vi "Fetch Measurement (Occupied Bandwidth).vi"(8 "error in (no error)":errorcluster, 9 "Timeout (20000 ms)":i32=20000, 11 "VISA resource name":refnum<visa-resource-name>) -> (0 "error out":errorcluster, 1 "Occupied Bandwidth (Hz)":dbl format="%#.6g", 2 "Transmit Frequency Error (Hz)":dbl format="%#.6g", 3 "VISA resource name out":refnum<visa-resource-name>, 5 "x dB Bandwidth (Hz)":dbl format="%#.6g")   [LabVIEW 2014, in "Agilent ESA PSA Series.lvlib"]
doc: "Returns the results of the last measurement(Occupied Bandwidth) and does not initiate data acquisition."
uses:
  Agilent ESA PSA Series.lvlib
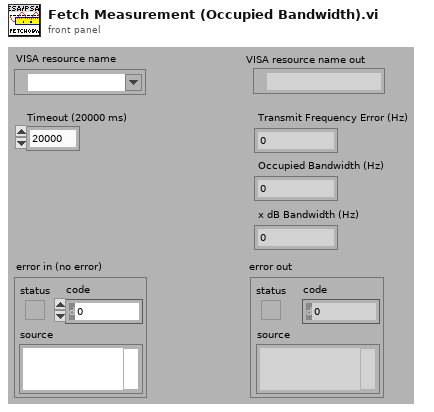
[diagram p1: front panel]
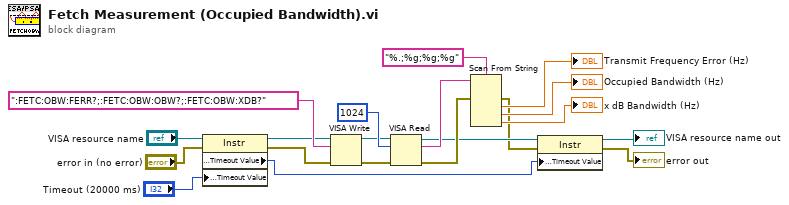
[diagram p0: block diagram]
diagram:
  n1 = property on="Property Node" class="Instr"(reference="VISA resource name", error in="error in (no error)", "General Settings:Timeout Value"="Timeout (20000 ms)") -> (reference out=w8:refnum<visa-resource-name>, error out=w7:errorcluster, "General Settings:Timeout Value"=w2:u32)
  n2 = VISA Write(VISA resource name=w8, write buffer=":FETC:OBW:FERR?;:FETC:OBW:OBW?;:FETC:OBW:XDB?" ("format string"), error in (no error)=w7) -> (VISA resource name out=w16:refnum<visa-resource-name>, error out=w15:errorcluster)  [unwired: 1 out]
  n3 = VISA Read(VISA resource name=w16, byte count=u32 1024, error in (no error)=w15) -> (VISA resource name out=w6:refnum<visa-resource-name>, read buffer=w19:string, error out=w18:errorcluster)  [unwired: 1 out]
  n4 = Scan From String(format string="%.;%g;%g;%g", input string=w19, error in=w18) -> (error out=w5:errorcluster, output 1=→"Transmit Frequency Error (Hz)":dbl, output 2=→"Occupied Bandwidth (Hz)":dbl, output 3=→"x dB Bandwidth (Hz)":dbl)  [unwired: 4 in, 2 out]
  n5 = property on="Property Node" class="Instr"(reference=w6, error in=w5, "General Settings:Timeout Value"=w2) -> (reference out=→"VISA resource name out":refnum<visa-resource-name>, error out=→"error out":errorcluster)
